vi "Append New Transactions.vi"(8 "error in (no error)":errorcluster, 10 "TransactionList.lvclass":refnum<class "TransactionList.lvclass">, 11 "Database in":refnum<class "Account History.lvclass">) -> (0 "error out":errorcluster, 1 "Num records":i32, 3 "Database out":refnum<class "Account History.lvclass">)   [LabVIEW 2018, in "Account History.lvclass"]
uses:
  Account History.lvclass
  Statement/TransactionList.lvclass
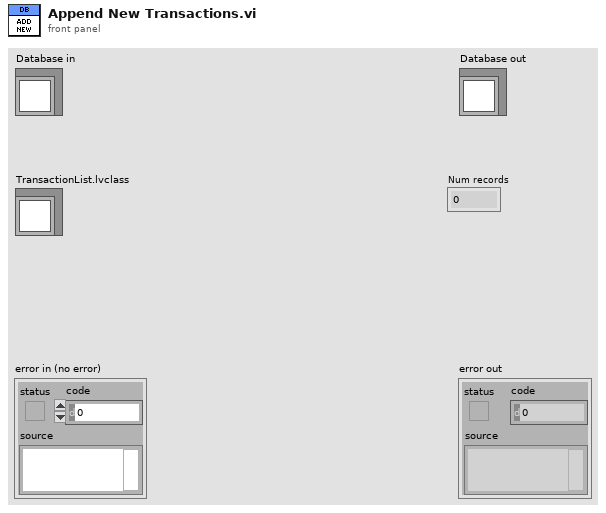
[diagram p1: front panel]
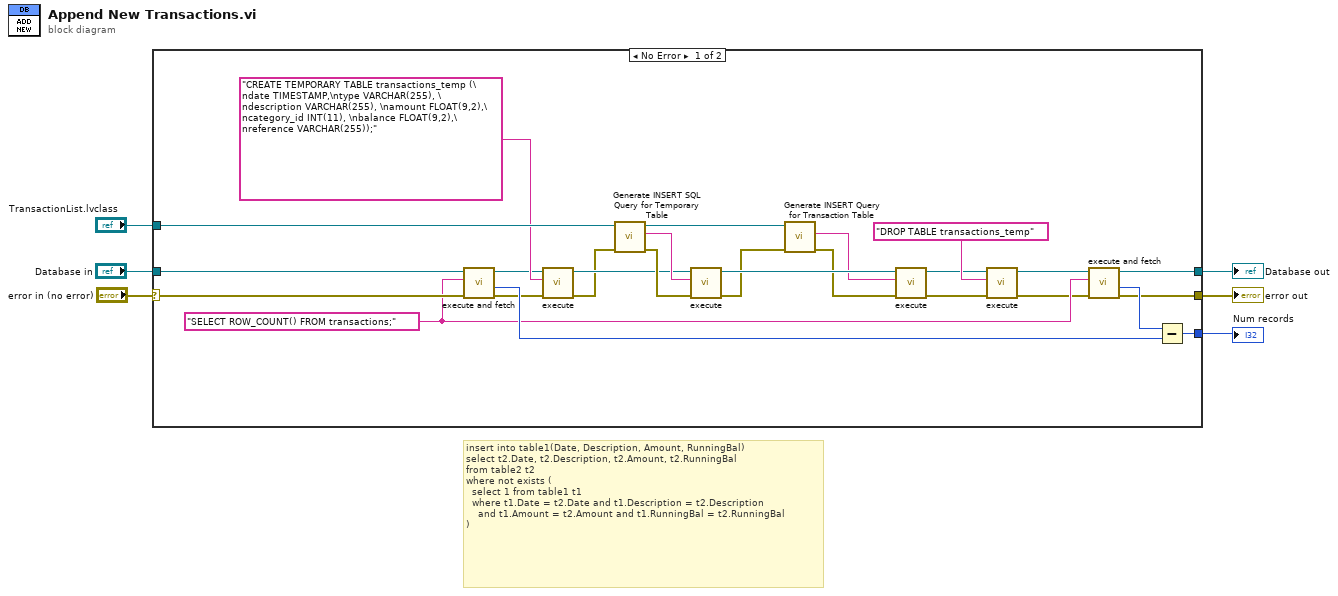
[diagram p0: block diagram]
diagram:
  # "insert into table1(Date, Description, Amount, RunningBal)\nselect t2.Date, t2.Description, t2.Amount, t2.RunningBal\nfrom table2 t2\nwhere not exists (\n  select 1 from table1 t1\n  where t1.Date = t2.Date and t1.Description = t2.Description\n    and t1.Amount = t2.Amount and t1.RunningBal = t2.RunningBal\n)"
  n1 = case shown="No Error" "error in (no error)" {
    selector: "error in (no error)" -> [w22 w33]
    tunnel: "Database in" -> [w23 w34]
    tunnel: [w13 w34] -> w5
    tunnel: [w12 w33] -> w4
    tunnel: "TransactionList.lvclass" -> [w32 _]
    tunnel: [w19 _] -> w2
    frame No Error {
      w11 = "SELECT ROW_COUNT() FROM transactions;" ("SQL query")
      n2 = call "execute and fetch.vi"("error in (no error)"=w22, "SQL query"=w11, "Database in"=w23) -> ("error out"=w15:errorcluster, "Num records"=w20:i32, "Database out"=w17:refnum<class "Account History.lvclass">)  [unwired: 5 in, 1 out]
      n3 = call "execute.vi"("error in (no error)"=w15, "SQL query"="CREATE TEMPORARY TABLE transactions_temp (\ndate TIMESTAMP,\ntype VARCHAR(255), \ndescription VARCHAR(255), \namount FLOAT(9,2),\ncategory_id INT(11), \nbalance FLOAT(9,2),\nreference VARCHAR(255));", "Database in"=w17) -> ("error out"=w14:errorcluster, "Database out"=w16:refnum<class "Account History.lvclass">)  [unwired: 7 in]
      n4 = call-dynamic "Generate INSERT SQL Query for Temporary Table.vi"("error in (no error)"=w14, "Importing Transactions"=w32) -> ("error out"=w28:errorcluster, "INSERT Query"=w29:string, "Statement.lvclass"=w27:refnum<class "TransactionList.lvclass">)  [unwired: 7 in]
      n5 = call "execute.vi"("error in (no error)"=w28, "SQL query"=w29, "Database in"=w16) -> ("error out"=w26:errorcluster, "Database out"=w30:refnum<class "Account History.lvclass">)  [unwired: 7 in]
      n6 = call-dynamic "Generate INSERT Query for Transaction Table.vi"("error in (no error)"=w26, "Statement in"=w27) -> ("error out"=w25:errorcluster, "Insert Query"=w24:string)  [unwired: 7 in, 1 out]
      n7 = call "execute.vi"("error in (no error)"=w25, "SQL query"=w24, "Database in"=w30) -> ("error out"=w9:errorcluster, "Database out"=w10:refnum<class "Account History.lvclass">)  [unwired: 7 in]
      n8 = call "execute.vi"("error in (no error)"=w9, "SQL query"="DROP TABLE transactions_temp", "Database in"=w10) -> ("error out"=w7:errorcluster, "Database out"=w8:refnum<class "Account History.lvclass">)  [unwired: 7 in]
      n9 = call "execute and fetch.vi"("error in (no error)"=w7, "SQL query"=w11, "Database in"=w8) -> ("error out"=w12:errorcluster, "Num records"=w21:i32, "Database out"=w13:refnum<class "Account History.lvclass">)  [unwired: 5 in, 1 out]
      n10 = Subtract(x=w21, y=w20) -> (x-y=w19:i32)
    }
    frame Error {
    }
  }
  "error out" <- w4
  "Database out" <- w5
  "Num records" <- w2
